vi "Update_DestDir_For_Main_Dest_Change.vi"(8 "error in (no error)":errorcluster, 11 "AB_Build in":refnum<class "AB_Build.lvclass">) -> (0 "error out":errorcluster, 3 "AB_Build out":refnum<class "AB_Build.lvclass">)   [LabVIEW 2020, in "AB_Build.lvclass"]
uses:
  <vilib>/AppBuilder/AB_Classes/Build/AB_Build.lvclass
  <vilib>/AppBuilder/AB_Classes/Build/AB_Build.lvclass/AB_Build.ctl
  <vilib>/AppBuilder/AB_Classes/Destination/AB_Destination.lvclass
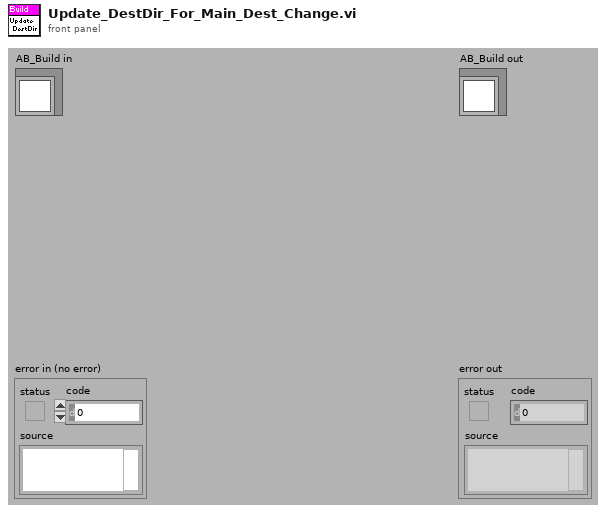
[diagram p1: front panel]
types:
  T1 = typedef "AB_Destination.ctl" = cluster{"destName":string, "path":path, "libraryName":string, "preserveHierarchy":bool, "eng_inBuild":bool, "eng_libraryReference":refnum<vi>, "eng_restictAddToNewLibrary":bool}
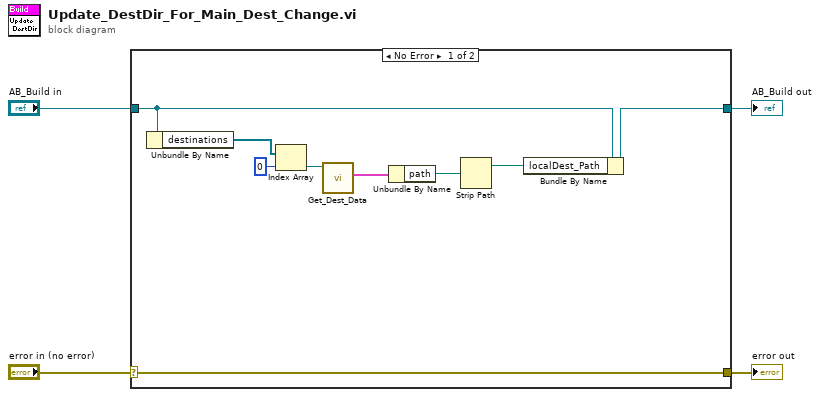
[diagram p0: block diagram]
diagram:
  n1 = case shown="No Error" "error in (no error)" {
    selector: "error in (no error)" -> [w13 w15]
    tunnel: [w13 w15] -> w3
    tunnel: [w12 w14] -> w1
    tunnel: "AB_Build in" -> [w11 w14]
    frame No Error {
      n2 = Unbundle By Name(w11) -> ("destinations"=w10:refnum<class "AB_Destination.lvclass">[])
      n3 = Index Array(array=w10, index=0) -> (element=w8:refnum<class "AB_Destination.lvclass">)
      n4 = call <vilib>:"Get_Dest_Data.vi"("Class in"=w8) -> ("destName"=w7:T1)  [unwired: 8 in, 2 out]
      n5 = Unbundle By Name(w7) -> ("path"=w6:path)
      n6 = Strip Path(path=w6) -> (stripped path=w5:path)  [unwired: 1 out]
      n7 = Bundle By Name(cluster=w11, "localDest_Path"=w5) -> (w12:refnum<class "AB_Build.lvclass">)
    }
    frame Error {
    }
  }
  "error out" <- w3
  "AB_Build out" <- w1
